vi "Window-Simple Time Series Player.vi"() -> ()   [LabVIEW 2017]
uses:
  User Interface/Visualisation/Timelapse Viewer/Typedefs/Custom slider-vertical.ctl
  User Interface/Visualisation/Timelapse Viewer/Typedefs/Time series viewer refs.ctl
  <vilib>/Utility/miscctls.llb/LVPointTypeDef.ctl
  User Interface/Visualisation/Timelapse Viewer/Typedefs/Speed Viewer States enum.ctl
  Typedefs/Save-Load enum.ctl
  Typedefs/HW config states enum.ctl
  User Interface/Visualisation/Functional Imaging Viewer/Typedefs/Get-Set-Clear Control.ctl
  User Interface/Visualisation/Timelapse Viewer/Typedefs/Select Play-Stop button to show.ctl
  <vilib>/vision/Image Controls.llb/IMAQ Image.ctl
  User Interface/Visualisation/Timelapse Viewer/Globals/gl_Time series viewer globals.vi
  Global Variables/General Globals.vi
panel:
  in  "Intensity":T1={-4095.0, 4095.0} scale=0.0..4095.0
  in  "Back":bool
  in  "Play":bool
  in  "Stop":bool
  in  "Colour":u16(ring)=2 items=["Gray", "Red", "Green"]
  out "Image":T2(plugin-control)
  in  "AVI File Path":path
  out "Speed Graph":dbl[](graph) caption="Speed Chart"
  out "Export data subset":bool
  out "Export vid":bool
  out "Stop (ind)":bool
  in  "Scrollbar":i32(c297)
  out "Speed Profile Graph":dbl[](graph)
  # "<-- Available through the menu"
  # "<-- Available through the menu"
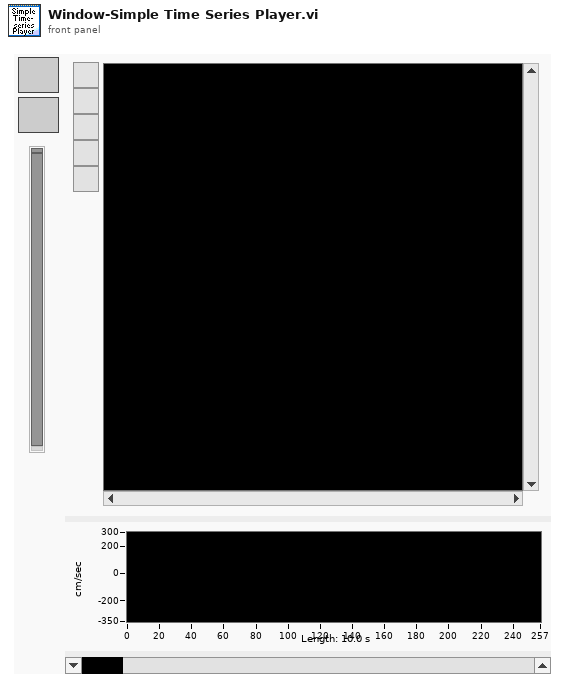
[diagram p1: front panel]
types:
  T1 = typedef "Custom slider-vertical.ctl" = cluster{dbl, dbl}
  T2 = typedef "IMAQ Image.ctl" = refnum<image>
  T3 = typedef "Time series viewer refs.ctl" = cluster{"This VI":refnum<vi>, "Image control":refnum<vi>, "AVI Mode ind":refnum<vi>, "Play":refnum<vi>, "Stop":refnum<vi>, "Back":refnum<vi>, "Scrollbar":refnum<vi>, "Video length info":refnum<vi>, "Expected speed values":refnum<vi>, "Intensity":refnum<vi>, "Path":refnum<vi>, "Selection sliders":refnum<vi>, "Speed Graph ref":refnum<vi>, "Frame rate set (fps)":refnum<vi>, "Channel to load":refnum<vi>, "Number of rows to generate":refnum<vi>, "Colour":refnum<vi>}
  T4 = typedef "LVPointTypeDef.ctl" = cluster{"Horizontal":i16, "Vertical":i16}
  T5 = typedef "HW config states enum.ctl" = enum16{"Load from file", "Save to file", "Write all", "Read all", "Write XY stage settings", "Write DAQ FPGA settings", "Write Control FPGA settings", "Write Phys Channels", "Write System Config", "Write HW Config", "Save System Config", "Save HW Config", "Clear", "Compare from file"}
  T6 = typedef "Save-Load enum.ctl" = enum16{"Save to file", "Load from file", "Compare from file"}
  T7 = typedef "Speed Viewer States enum.ctl" = enum16{"Idle", "Initialise", "Playback", "Scroll bar event", "Speed cursor event", "Back to start", "Exit"}
  T8 = typedef "Image Type" = u32
  T9 = typedef "Custom slider-horisontal.ctl" = cluster{dbl, dbl}
  T10 = typedef "Select Play-Stop button to show.ctl" = enum16{"Show Play button", "Show Stop button"}
  T11 = typedef "AVI modes refs cluster.ctl" = cluster{"AVI1 ref":T12, "AVI2 refs":T13[], "AVI # frames":u32[]}
  T12 = typedef "AviRefnum.ctl" = refnum<k1>
  T13 = typedef "IMAQ AVI2 Refnum.ctl" = refnum<k20>
  T14 = typedef "AVI implementation enum.ctl" = enum16{"AVI1", "AVI2"}
  T15 = cluster{"# of frames to export":i32, "Initial frame's owning file":T13, "8-bit AVI file path":path, "Cursors location":cluster{"Number of first frame":i32, "Number of last frame":i32}}
  T16 = typedef "Get-Set-Clear Control.ctl" = enum16{"Get", "Set", "Clear"}
  T17 = typedef "Speed graph behaviour enum.ctl" = enum16{"Scrolling data", "Scrolling cursor"}
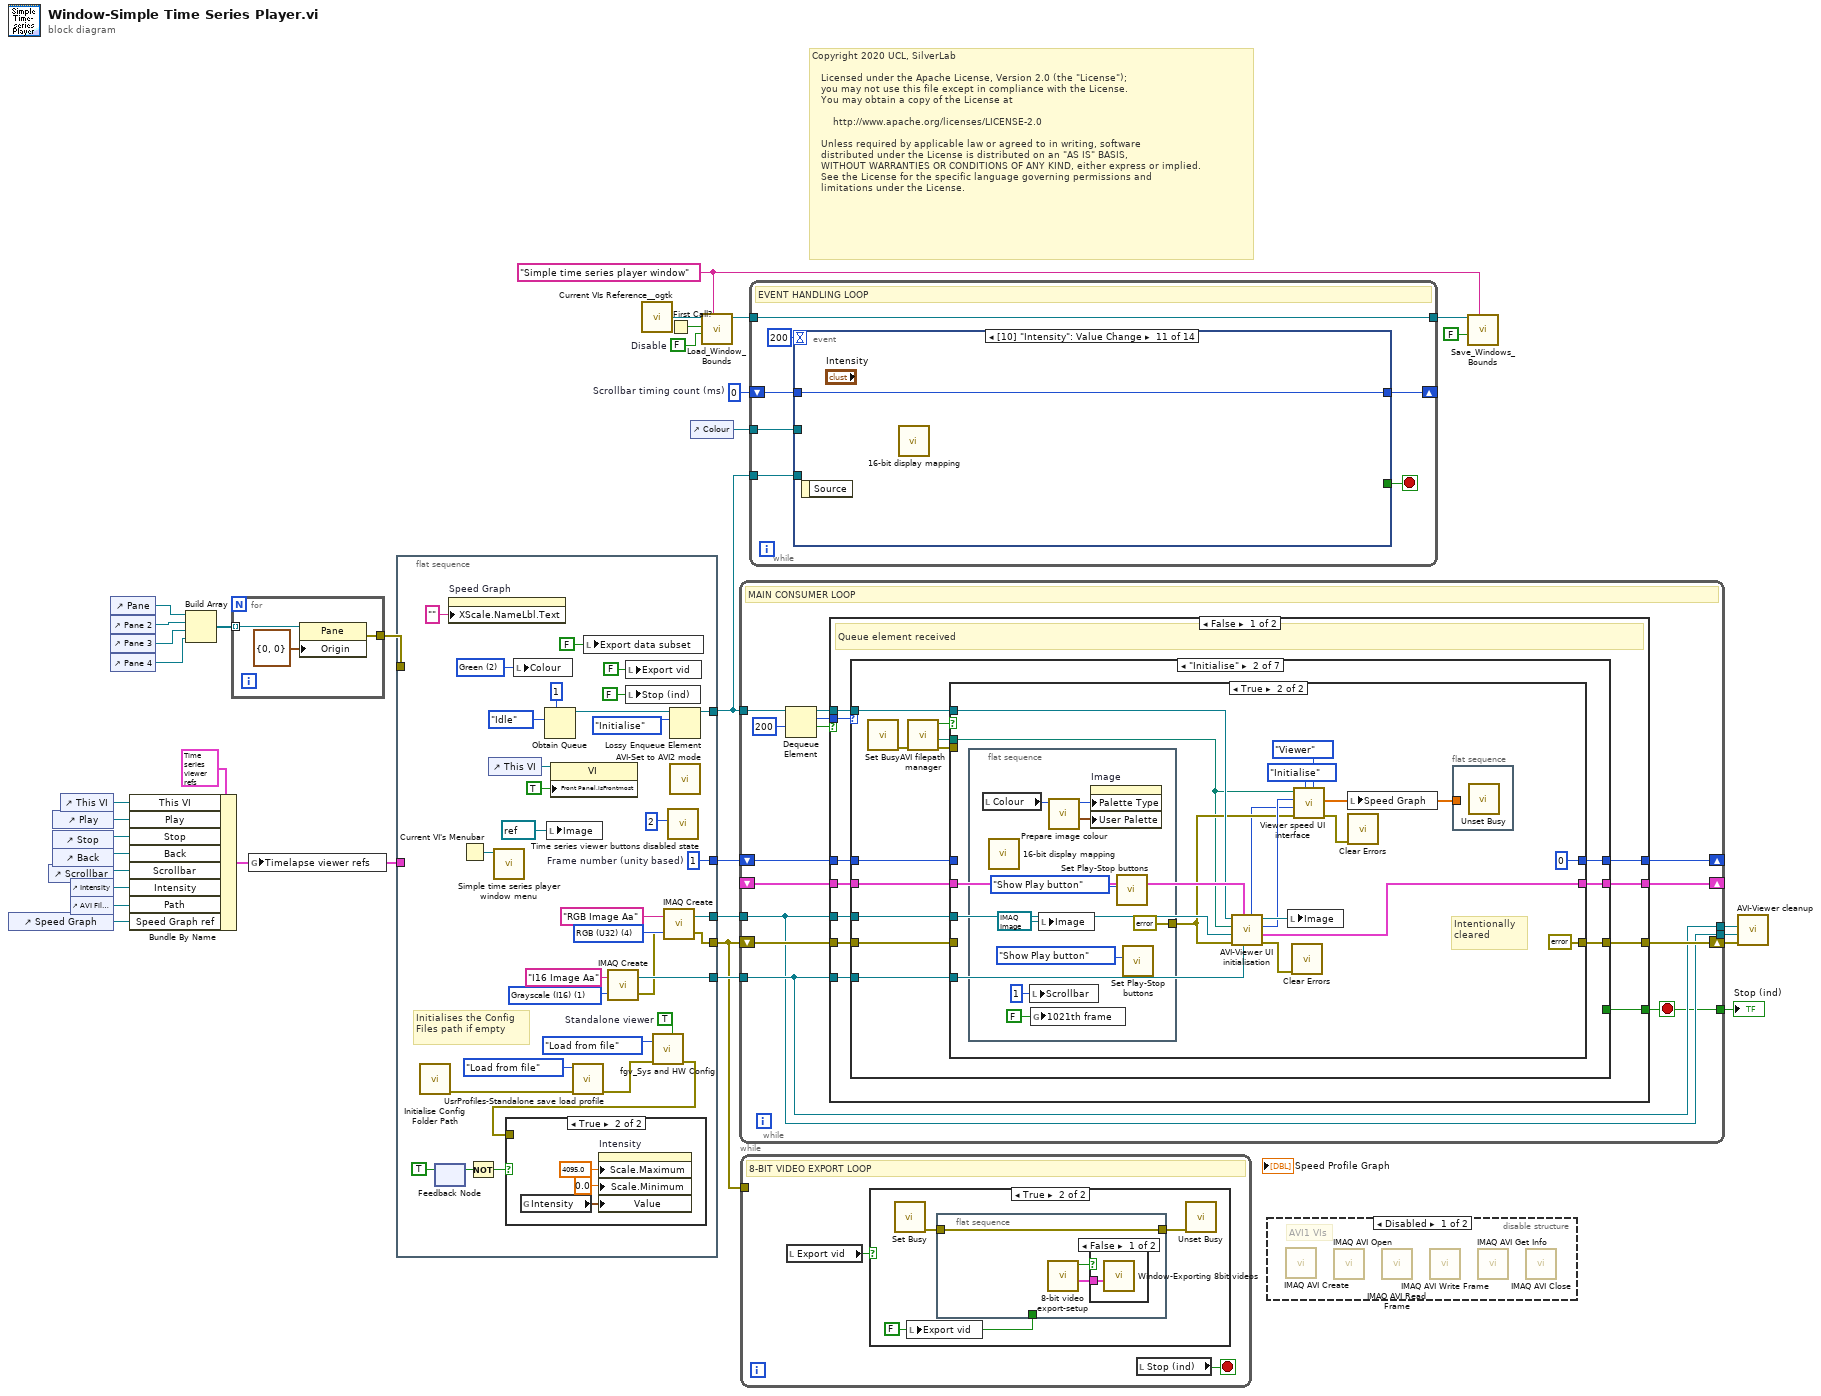
[diagram p0: block diagram]
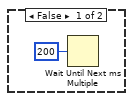
[diagram p3: hidden frame]
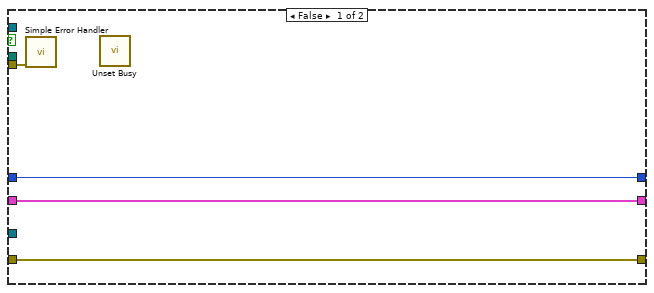
[diagram p7: hidden frame]
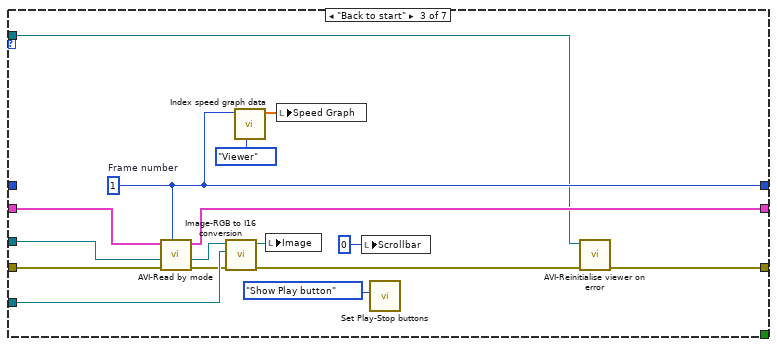
[diagram p8: hidden frame]
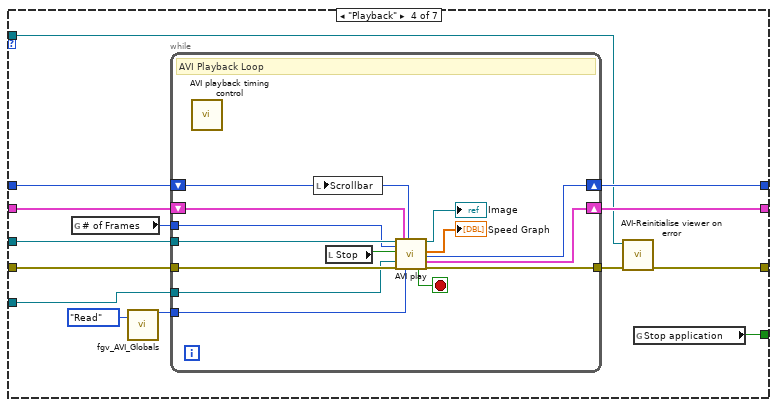
[diagram p9: hidden frame]
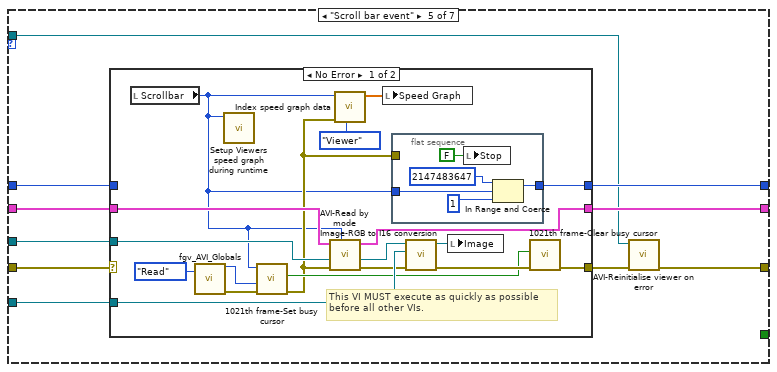
[diagram p10: hidden frame]
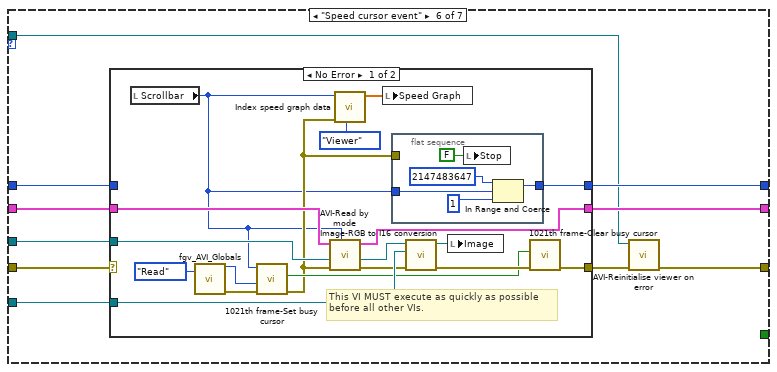
[diagram p12: hidden frame]
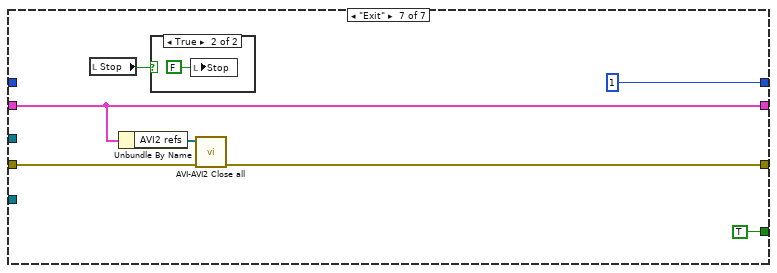
[diagram p14: hidden frame]
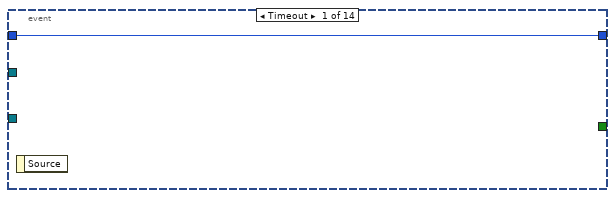
[diagram p17: hidden frame]
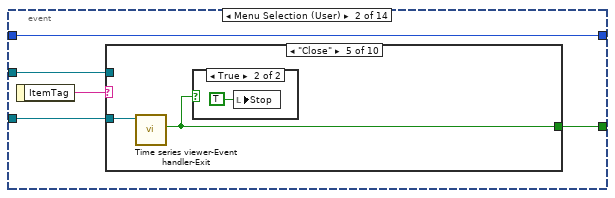
[diagram p18: hidden frame]
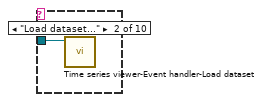
[diagram p20: hidden frame]
diagram:
  w6 = FALSE  # Disable
  w5 = "Simple time series player window" ("Window Name (i.e. Key)")
  w22 = u32 0  # Scrollbar timing count (ms)
  # "Copyright 2020 UCL, SilverLab\n \n   Licensed under the Apache License, Version 2.0 (the \"License\");\n   you may not use this file except in compliance with the License.\n   You may obtain a copy of the License at\n \n       http://www.apache.org/licenses/LICENSE-2.0\n \n   Unless required by applicable law or agreed to in writing, software\n   distributed under the License is distributed on an \"AS IS\" BASIS,\n   WITHOUT WARRANTIES OR CONDITIONS OF ANY KIND, either express or implied.\n   See the License for the specific language governing permissions and\n   limitations under the License."
  n1 = control-ref of="Speed Graph"() -> (w1:refnum<vi>)
  n2 = control-ref of="Scrollbar"() -> (w24:refnum<vi>)
  n3 = control-ref of="Play"() -> (w27:refnum<vi>)
  n4 = control-ref of="Stop"() -> (w26:refnum<vi>)
  n5 = control-ref of="Back"() -> (w25:refnum<vi>)
  n6 = control-ref of="This VI"() -> (w16:refnum<vi>)
  n7 = control-ref of="Intensity"() -> (w23:refnum<vi>)
  n8 = control-ref of="AVI File Path"() -> (w21:refnum<vi>)
  n9 = control-ref of="Pane"() -> (w14:refnum<vi>)
  n10 = control-ref of="Pane 2"() -> (w13:refnum<vi>)
  n11 = control-ref of="Pane 3"() -> (w12:refnum<vi>)
  n12 = control-ref of="Pane 4"() -> (w11:refnum<vi>)
  n13 = Bundle By Name(cluster=T3 {"This VI"=refnum, "Image control"=refnum, "AVI Mode ind"=refnum, "Play"=refnum, "Stop"=refnum, "Back"=refnum, "Scrollbar"=refnum, "Video length info"=refnum, "Expected speed values"=refnum, "Intensity"=refnum, "Path"=refnum, "Selection sliders"=refnum, "Speed Graph ref"=refnum, "Frame rate set (fps)"=refnum, "Channel to load"=refnum, "Number of rows to generate"=refnum, "Colour"=refnum}, "This VI"=w16, "Play"=w27, "Stop"=w26, "Back"=w25, "Scrollbar"=w24, "Intensity"=w23, "Path"=w21, "Speed Graph ref"=w1) -> (w19:T3)
  n14 = Build Array(w14, w13, w12, w11) -> (w10:refnum<vi>[])
  n15 = for {
    tunnel: w10 -> [w36] mode=indexing
    tunnel: [w35] -> w9
    n16 = property class="Pane"(reference=w36, "Origin"=T4 {"Horizontal"=0, "Vertical"=0}) -> (error out=w35:errorcluster)  [unwired: 1 in, 1 out]
  }
  n17 = global write "gl_Time series viewer globals.vi" "Timelapse viewer refs"(w19) -> ()
  n18 = flat-sequence {
    tunnel: [w68] -> w34
    tunnel: [w65] -> w33
    tunnel: [w57] -> w17
    tunnel: [w61] -> w31
    tunnel: [w59] -> w30
    tunnel: w19 -> [_]
    tunnel: w9 -> [_]
    frame #0 {
      w38 = TRUE  # Standalone viewer
      w50 = u16 2 items=["Gray", "Red", "Green"] ("Colour")
      w59 = 1  # Frame number (unity based)
      w67 = T8 1 items=["Grayscale (U8)", "Grayscale (I16)", "Grayscale (SGL)", "Complex (CSG)", "RGB (U32)", "HSL (U32)", "RGB (U64)", "Grayscale (U16)"] ("Image Type")
      w69 = T8 4 items=["Grayscale (U8)", "Grayscale (I16)", "Grayscale (SGL)", "Complex (CSG)", "RGB (U32)", "HSL (U32)", "RGB (U64)", "Grayscale (U16)"] ("Image Type")
      # "Initialises the Config Files path if empty"
      n19 = call "Initialise Config Folder Path.vi"() -> ("error out"=w46:errorcluster)  [unwired: 9 in, 2 out]
      n20 = feedback #1() -> (w43:bool)  [unwired: 1 in]
      n21 = feedback-in #1(TRUE) -> ()
      n22 = property on="Speed Graph" class="WFGraph (strict)"("XScale.NameLbl.Text"="" ("X Scale.Name Label.Text")) -> ()  [unwired: 2 in, 2 out]
      n23 = Current VI's Menubar() -> (w51:refnum<k9>)
      n24 = Not(x=w43) -> (.not. x?=w45:bool)
      n25 = control-ref of="This VI"() -> (w55:refnum<vi>)
      n26 = call "Simple time series player window menu.vi"("menu"=w51) -> ()  [unwired: 9 in, 2 out]
      n27 = local write "Colour"(w50) -> ()
      n28 = Obtain Queue(max queue size (-1, unlimited)=1, element data type=Speed_Viewer_States_enum."Idle" ("States")) -> (queue out=w62:refnum<queue>)  [unwired: 3 in, 2 out]
      n29 = local write "Image"(refnum<image> refnum ("New Image")) -> ()
      n30 = property on="Property Node" class="VI"(reference=w55, "Front Panel.IsFrontmost"=TRUE ("Front Panel Window:Is Frontmost")) -> ()  [unwired: 1 in, 2 out]
      n31 = call "UsrProfiles-Standalone save load profile.vi"("Error in"=w46, "Function"=Save-Load_enum."Load from file") -> ("error out"=w40:errorcluster)  [unwired: 9 in]
      n32 = local write "Export data subset"(FALSE ("Export data subset")) -> ()
      n33 = call "IMAQ Create"("Image Name"="I16 Image Aa", "Image Type"=w67) -> ("New Image"=w65:T2, "error out"=w58:errorcluster)  [unwired: 2 in, 1 out]
      n34 = local write "Export vid"(FALSE ("Export")) -> ()
      n35 = local write "Stop (ind)"(FALSE ("Boolean")) -> ()
      n36 = call "fgv_Sys and HW Config.vi"("Standalone viewer initialisation?"=w38, "Function"=HW_config_states_enum."Load from file", "error in (no error)"=w40) -> ("error out"=w39:errorcluster)  [unwired: 6 in, 2 out]
      n37 = case shown="True" w45 {
        tunnel: w39 -> [_ _]
        frame False {
        }
        frame True {
          n38 = global read "gl_Time series viewer globals.vi" "Intensity"() -> (w71:T9)
          n39 = property on="Intensity" class="Slide (strict)"("Scale.Maximum"=4095.0 ("Scale.Range:Maximum"), "Scale.Minimum"=0.0 ("Scale.Range:Minimum"), "Value"=w71) -> ()  [unwired: 2 in, 2 out]
        }
      }
      n40 = call "IMAQ Create"("Image Name"="RGB Image Aa", "Image Type"=w69, "error in (no error)"=w58) -> ("New Image"=w68:T2, "error out"=w57:errorcluster)  [unwired: 1 in, 1 out]
      n41 = call "Time series viewer buttons disabled state.vi"("Disabled"=2) -> ()  [unwired: 10 in, 1 out]
      n42 = Lossy Enqueue Element(queue=w62, element=Speed_Viewer_States_enum."Initialise" ("States")) -> (queue out=w61:refnum<queue>)  [unwired: 1 in, 3 out]
      n43 = call "AVI-Set to AVI2 mode.vi"() -> ()  [unwired: 11 in, 1 out]
    }
  }
  n44 = call <userlib>:"Current VIs Reference__ogtk.vi"() -> ("Current VI's reference"=w8:refnum<vi>)  [unwired: 5 in]
  n45 = First Call?() -> (First Call?: T/F=w7:bool)
  n46 = control-ref of="Colour"() -> (w15:refnum<vi>)
  n47 = call "Load_Window_Bounds.vi"("Window Name (i.e. Key)"=w5, "Disable"=w6, "First Call"=w7, "Window VI's Ref"=w8) -> ("reference out"=w3:refnum<vi>)  [unwired: 4 in, 3 out]
  n48 = while {
    tunnel: w34 -> [w76]
    tunnel: w33 -> [w77]
    tunnel: [w77] -> w32
    shift-right: [w84] -> _
    shift-left: w30 -> [w83]
    tunnel: w31 -> [w82]
    shift-right: [w78] -> _
    shift-left: _ -> [w87]
    tunnel: [w76] -> w20
    shift-right: [w85] -> w28
    shift-left: w17 -> [w86]
    tunnel: [w74] -> w18
    stop <- w74 stop-if-true
    # "MAIN CONSUMER LOOP"
    n49 = Dequeue Element(queue=w82, timeout in ms (-1)=200) -> (queue out=w75:refnum<queue>, element=w79:T7, timed out?=w80:bool)  [unwired: 1 in, 1 out]
    n50 = case shown="False" w80 {
      tunnel: w87 -> [w98 w270]
      tunnel: [w97 w270] -> w78
      tunnel: w76 -> [w96 _]
      tunnel: w77 -> [w95 _]
      tunnel: w86 -> [w94 w269]
      tunnel: [w93 w269] -> w85
      tunnel: [w92 w271] -> w84
      tunnel: w83 -> [w91 w271]
      tunnel: w79 -> [w90 _]
      tunnel: [w89 _] -> w74
      tunnel: w75 -> [w88 _]
      frame False {
        # "Queue element received"
        n51 = case shown="\"Initialise\"" w90 {
          tunnel: w98 -> [w100 w114 w158 w174 w194 w230 w263]
          tunnel: [w100 w110 w157 w168 w196 w232 w263] -> w97
          tunnel: w96 -> [_ w109 w155 w173 w195 w231 _]
          tunnel: w95 -> [_ w108 w156 w172 w198 w234 _]
          tunnel: w94 -> [w99 w112 w153 w171 w193 w229 w262]
          tunnel: [w99 w111 w148 w167 w191 w227 w261] -> w93
          tunnel: [w101 w113 w150 w170 w197 w233 1 ("Slide")] -> w92
          tunnel: w91 -> [w101 w107 _ w169 w192 w228 _]
          tunnel: [_ _ _ w161 _ _ TRUE] -> w89
          tunnel: w88 -> [_ w103 w147 w165 w189 w225 _]
          frame Default {
          }
          frame "Initialise" {
            n52 = call <vilib>:"Set Busy.vi"() -> ("error out"=w102:errorcluster)  [unwired: 10 in, 1 out]
            n53 = call "AVI filepath manager.vi"("error in (no error)"=w102) -> ("error"=w104:errorcluster, "AVI File Path"=w105:path, "File path OK"=w106:bool)  [unwired: 8 in]
            n54 = case shown="True" w106 {
              tunnel: w114 -> [w117 w135]
              tunnel: [w118 0] -> w113
              tunnel: w105 -> [_ w125]
              tunnel: w112 -> [w116 _]
              tunnel: [w116 errorcluster {"status"=FALSE, "code"=0, "source"=""} ("error out")] -> w111
              tunnel: [w117 w128] -> w110
              tunnel: w109 -> [_ w127]
              tunnel: w108 -> [_ w133]
              tunnel: w107 -> [w118 _]
              tunnel: w104 -> [w115 _]
              tunnel: w103 -> [_ w131]
              frame False {
                n55 = call <vilib>:"Simple Error Handler.vi"("error in (no error)"=w115) -> ()  [unwired: 4 in, 5 out]
                n56 = call <vilib>:"Unset Busy.vi"() -> ()  [unwired: 11 in, 1 out]
              }
              frame True {
                # "Intentionally cleared"
                n57 = flat-sequence {
                  tunnel: [errorcluster {"status"=FALSE, "code"=0, "source"=""} ("error out")] -> w126
                  frame #0 {
                    n58 = local read "Colour"() -> (w139:u16)
                    n59 = call "16-bit display mapping.vi"() -> ()  [unwired: 11 in, 1 out]
                    n60 = local write "Scrollbar"(1 ("Scrollbar")) -> ()
                    n61 = global write "gl_Time series viewer globals.vi" "1021th frame"(FALSE ("1021th frame")) -> ()
                    n62 = local write "Image"(T2 refnum ("New Image")) -> ()
                    n63 = call "Prepare image colour.vi"("Left Image Palette"=w139) -> ("Color Palette"=w141:cluster{"Red":u8, "Green":u8, "Blue":u8}[], "Palette Type"=w140:u32)  [unwired: 8 in, 1 out]
                    n64 = property on="Image" class="ImageControl"("Palette Type"=w140, "User Palette"=w141) -> ()  [unwired: 2 in, 2 out]
                    n65 = call "Set Play-Stop buttons.vi"("Function"=Select_Play-Stop_button_to_show."Show Play button") -> ()  [unwired: 10 in, 1 out]
                    n66 = call "Set Play-Stop buttons.vi"("Function"=Select_Play-Stop_button_to_show."Show Play button") -> ()  [unwired: 10 in, 1 out]
                  }
                }
                n67 = call "AVI-Viewer UI initialisation.vi"("I16 image ref in"=w133, "AVI modes refs in"=w135, "error in (no error)"=w126, "RGB image ref in"=w127, "AVI File Path"=w125, "Queue in"=w131) -> ("error out"=w120:errorcluster, "AVI modes refs out"=w128:T11, "Number of Frames"=w129:u32, "Refnum out"=w130:T2, "Scrollbar position"=w122:i32)  [unwired: 1 in]
                n68 = local write "Image"(w130) -> ()
                n69 = call <vilib>:"Clear Errors.vi"("error in (no error)"=w120) -> ()  [unwired: 5 in, 2 out]
                n70 = call "Viewer speed UI interface.vi"("Caller"=enum16{"Viewer", "Exporter"}."Viewer", "Function"=enum16{"Initialise", "Update"}."Initialise", "error in (no error)"=w126, "Gobal frame number in Timelapse data/master video (1 based)"=w122, "Number of Frames"=w129, "Speed Data folder path+dummy filename"=w125) -> ("error out"=w124:errorcluster, "Speed waveform graph data"=w119:dbl[])  [unwired: 2 in, 2 out]
                n71 = local write "Speed Graph"(w119) -> ()
                n72 = call <vilib>:"Clear Errors.vi"("error in (no error)"=w124) -> ()  [unwired: 5 in, 2 out]
                n73 = flat-sequence {
                  tunnel: w119 -> [_]
                  frame #0 {
                    n74 = call <vilib>:"Unset Busy.vi"() -> ()  [unwired: 11 in, 1 out]
                  }
                }
              }
            }
          }
          frame "Back to start" {
            w150 = 1  # Frame number
            n75 = call "AVI-Read by mode.vi"("Frame number (unity-based)"=w150, "error in (no error)"=w153, "RGB image ref in"=w155, "AVI modes refs"=w158) -> ("error out"=w152:errorcluster, "RGB image ref out"=w159:T2, "AVI modes refs"=w157:T11)  [unwired: 5 in]
            n76 = call "Image-RGB to I16 conversion.vi"("error in (no error)"=w152, "I16 image ref in"=w156, "RGB image ref in"=w159) -> ("error out"=w149:errorcluster, "I16 image ref out"=w154:T2)  [unwired: 7 in]
            n77 = call "Index speed graph data.vi"("Caller"=enum16{"Viewer", "Exporter"}."Viewer", "Gobal frame number in Timelapse data/master video (1 based)"=w150) -> ("Speed data waveform graph"=w145:dbl[])  [unwired: 7 in, 2 out]
            n78 = local write "Image"(w154) -> ()
            n79 = local write "Speed Graph"(w145) -> ()
            n80 = local write "Scrollbar"(0 ("Scrollbar")) -> ()
            n81 = call "Set Play-Stop buttons.vi"("Function"=Select_Play-Stop_button_to_show."Show Play button") -> ()  [unwired: 10 in, 1 out]
            n82 = call "AVI-Reinitialise viewer on error.vi"("error in (no error)"=w149, "Queue in"=w147) -> ("error out"=w148:errorcluster)  [unwired: 9 in]
          }
          frame "Playback" {
            n83 = global read "gl_Time series viewer globals.vi" "# of Frames"() -> (w162:u32)
            n84 = call "fgv_AVI_Globals.vi"("Function"=enum16{"Intialize", "Write", "Read", "Clear"}."Read") -> ("AVI mode"=w163:T14)  [unwired: 11 in, 3 out]
            n85 = while {
              tunnel: w173 -> [w186]
              tunnel: w172 -> [w178]
              tunnel: w171 -> [w184]
              tunnel: [w185] -> w166
              shift-right: [w182] -> w170
              shift-left: w169 -> [w183]
              shift-right: [w187] -> w168
              shift-left: w174 -> [w188]
              tunnel: w163 -> [w180]
              tunnel: w162 -> [w177]
              stop <- w181 stop-if-true
              # "AVI Playback Loop"
              n86 = call "AVI playback timing control.vi"() -> ()  [unwired: 8 in, 4 out]
              n87 = local write "Scrollbar"(w183) -> ()
              n88 = local read "Stop"() -> (w179:bool)
              n89 = call "AVI play.vi"("RGB Image ref"=w186, "Number of Frames"=w177, "Stop button pressed"=w179, "I16 Image ref"=w178, "error in (no error)"=w184, "AVI modes refs in"=w188, "AVI mode"=w180, "Frame number (in)"=w183) -> ("Playback stopped"=w181:bool, "I16 image ref out"=→"Image":T2, "Speed data waveform graph"=→"Speed Graph":dbl[], "Frame number (out)"=w182:i32, "AVI modes refs out"=w187:T11, "error out"=w185:errorcluster)  [unwired: 6 in]
            }
            n90 = call "AVI-Reinitialise viewer on error.vi"("error in (no error)"=w166, "Queue in"=w165) -> ("error out"=w167:errorcluster)  [unwired: 9 in]
            n91 = global read "General Globals.vi" "Stop application"() -> (w161:bool)
          }
          frame "Scroll bar event" {
            n92 = case shown="No Error" w193 {
              selector: w193 -> [_ w224]
              tunnel: w198 -> [w216 _]
              tunnel: [w214 w223] -> w197
              tunnel: [w203 w222] -> w196
              tunnel: w195 -> [w212 _]
              tunnel: w194 -> [w210 w222]
              tunnel: [w205 w224] -> w190
              tunnel: w192 -> [_ w223]
              frame No Error {
                # "This VI MUST execute as quickly as possible\nbefore all other VIs."
                n93 = local read "Scrollbar"() -> (w199:i32)
                n94 = call "fgv_AVI_Globals.vi"("Function"=enum16{"Intialize", "Write", "Read", "Clear"}."Read") -> ("AVI mode"=w208:T14, "error out"=w207:errorcluster)  [unwired: 11 in, 2 out]
                n95 = call "Setup Viewers speed graph during runtime.vi"("Frame number or cycle number"=w199) -> ()  [unwired: 10 in, 1 out]
                n96 = call "1021th frame-Set busy cursor.vi"("error in (no error)"=w207, "AVI mode"=w208, "Frame number"=w199) -> ("error out"=w202:errorcluster, "Busy cursor was set"=w204:bool)  [unwired: 7 in]
                n97 = call "AVI-Read by mode.vi"("Frame number (unity-based)"=w199, "error in (no error)"=w202, "RGB image ref in"=w212, "AVI modes refs"=w210) -> ("error out"=w213:errorcluster, "RGB image ref out"=w211:T2, "AVI modes refs"=w203:T11)  [unwired: 5 in]
                n98 = call "Index speed graph data.vi"("Caller"=enum16{"Viewer", "Exporter"}."Viewer", "error in (no error)"=w202, "Gobal frame number in Timelapse data/master video (1 based)"=w199) -> ("Speed data waveform graph"=w200:dbl[])  [unwired: 6 in, 2 out]
                n99 = local write "Speed Graph"(w200) -> ()
                n100 = flat-sequence {
                  tunnel: [w219] -> w214
                  tunnel: w199 -> [w217]
                  tunnel: w202 -> [_]
                  frame #0 {
                    n101 = local write "Stop"(FALSE ("Stop")) -> ()
                    n102 = In Range and Coerce(upper limit=2147483647, x=w217, lower limit=1) -> (coerced(x)=w219:i32)  [unwired: 1 out]
                  }
                }
                n103 = call "Image-RGB to I16 conversion.vi"("error in (no error)"=w213, "I16 image ref in"=w216, "RGB image ref in"=w211) -> ("error out"=w206:errorcluster, "I16 image ref out"=w215:T2)  [unwired: 7 in]
                n104 = local write "Image"(w215) -> ()
                n105 = call "1021th frame-Clear busy cursor.vi"("error in (no error)"=w206, "Busy cursor was set"=w204) -> ("error out"=w205:errorcluster)  [unwired: 9 in]
              }
              frame Error {
              }
            }
            n106 = call "AVI-Reinitialise viewer on error.vi"("error in (no error)"=w190, "Queue in"=w189) -> ("error out"=w191:errorcluster)  [unwired: 9 in]
          }
          frame "Speed cursor event" {
            n107 = case shown="No Error" w229 {
              selector: w229 -> [_ w260]
              tunnel: w234 -> [w252 _]
              tunnel: [w250 w259] -> w233
              tunnel: [w239 w258] -> w232
              tunnel: w231 -> [w248 _]
              tunnel: w230 -> [w246 w258]
              tunnel: [w241 w260] -> w226
              tunnel: w228 -> [_ w259]
              frame No Error {
                # "This VI MUST execute as quickly as possible\nbefore all other VIs."
                n108 = local read "Scrollbar"() -> (w235:i32)
                n109 = call "fgv_AVI_Globals.vi"("Function"=enum16{"Intialize", "Write", "Read", "Clear"}."Read") -> ("AVI mode"=w244:T14, "error out"=w243:errorcluster)  [unwired: 11 in, 2 out]
                n110 = call "1021th frame-Set busy cursor.vi"("error in (no error)"=w243, "AVI mode"=w244, "Frame number"=w235) -> ("error out"=w238:errorcluster, "Busy cursor was set"=w240:bool)  [unwired: 7 in]
                n111 = call "AVI-Read by mode.vi"("Frame number (unity-based)"=w235, "error in (no error)"=w238, "RGB image ref in"=w248, "AVI modes refs"=w246) -> ("error out"=w249:errorcluster, "RGB image ref out"=w247:T2, "AVI modes refs"=w239:T11)  [unwired: 5 in]
                n112 = call "Index speed graph data.vi"("Caller"=enum16{"Viewer", "Exporter"}."Viewer", "error in (no error)"=w238, "Gobal frame number in Timelapse data/master video (1 based)"=w235) -> ("Speed data waveform graph"=w236:dbl[])  [unwired: 6 in, 2 out]
                n113 = local write "Speed Graph"(w236) -> ()
                n114 = flat-sequence {
                  tunnel: [w255] -> w250
                  tunnel: w235 -> [w253]
                  tunnel: w238 -> [_]
                  frame #0 {
                    n115 = local write "Stop"(FALSE ("Stop")) -> ()
                    n116 = In Range and Coerce(upper limit=2147483647, x=w253, lower limit=1) -> (coerced(x)=w255:i32)  [unwired: 1 out]
                  }
                }
                n117 = call "Image-RGB to I16 conversion.vi"("error in (no error)"=w249, "I16 image ref in"=w252, "RGB image ref in"=w247) -> ("error out"=w242:errorcluster, "I16 image ref out"=w251:T2)  [unwired: 7 in]
                n118 = local write "Image"(w251) -> ()
                n119 = call "1021th frame-Clear busy cursor.vi"("error in (no error)"=w242, "Busy cursor was set"=w240) -> ("error out"=w241:errorcluster)  [unwired: 9 in]
              }
              frame Error {
              }
            }
            n120 = call "AVI-Reinitialise viewer on error.vi"("error in (no error)"=w226, "Queue in"=w225) -> ("error out"=w227:errorcluster)  [unwired: 9 in]
          }
          frame "Exit" {
            n121 = local read "Stop"() -> (w267:bool)
            n122 = Unbundle By Name(w263) -> ("AVI2 refs"=w264:T13[])
            n123 = case shown="True" w267 {
              frame False {
              }
              frame True {
                n124 = local write "Stop"(FALSE ("Stop")) -> ()
              }
            }
            n125 = call "AVI-AVI2 Close all.vi"("error in (no error)"=w262, "AVI2 ref"=w264) -> ("error out"=w261:errorcluster)  [unwired: 9 in]
          }
        }
      }
      frame True {
        # "Timeout"
      }
    }
  }
  "Stop (ind)" <- w18
  n126 = while {
    tunnel: w17 -> [_]
    stop <- w273 stop-if-true
    # "8-BIT VIDEO EXPORT LOOP"
    n127 = local read "Export vid"() -> (w272:bool)
    n128 = case shown="True" w272 {
      frame False {
        n129 = Wait Until Next ms Multiple(millisecond multiple=u32 200) -> ()  [unwired: 1 out]
      }
      frame True {
        w277 = FALSE ("Export")
        n130 = call <vilib>:"Set Busy.vi"() -> ("error out"=w276:errorcluster)  [unwired: 10 in, 1 out]
        n131 = local write "Export vid"(w277) -> ()
        n132 = flat-sequence {
          tunnel: w277 -> [_]
          tunnel: w276 -> [w280]
          tunnel: [w280] -> w275
          frame #0 {
            n133 = call "8-bit video export-setup.vi"() -> ("output cluster"=w278:T15, "cancelled"=w279:bool)  [unwired: 9 in, 1 out]
            n134 = case shown="False" w279 {
              tunnel: w278 -> [w281 _]
              frame False {
                n135 = call "Window-Exporting 8bit videos.vi"("Input cluster"=w281) -> ()  [unwired: 11 in]
              }
              frame True {
              }
            }
          }
        }
        n136 = call <vilib>:"Unset Busy.vi"("error in (no error)"=w275) -> ()  [unwired: 10 in, 1 out]
      }
    }
    n137 = local read "Stop (ind)"() -> (w273:bool)
  }
  n138 = while {
    shift-right: [w286] -> _
    shift-left: w22 -> [w285]
    tunnel: w31 -> [w284]
    tunnel: w15 -> [w283]
    tunnel: [w282] -> w2
    tunnel: w3 -> [w282]
    stop <- w287 stop-if-true
    # "EVENT HANDLING LOOP"
    n139 = event shown="[10] \"Intensity\": Value Change" {
      selector: _ -> [_ _ _ _ _ _ _ _ _ _ _ _ _ _]
      dyn-events: _ -> [_ _ _ _ _ _ _ _ _ _ _ _ _ _]
      timeout: 200 -> [_ _ _ _ _ _ _ _ _ _ _ _ _ _]
      tunnel: [_ w291 _ _ _ _ _ _ _ _ _ _ _ w360] -> w287
      tunnel: [w289 w294 w309 w310 w318 w326 w330 w336 w339 w345 w346 w350 w358 w362] -> w286
      tunnel: w285 -> [w289 w294 w309 w312 w318 w326 w330 w336 w339 w345 w346 w350 w358 w362]
      tunnel: w284 -> [_ w292 _ w311 _ w324 _ _ w338 w342 _ w349 _ w361]
      tunnel: w283 -> [_ w290 _ _ _ _ _ _ _ _ _ _ _ _]
      event Timeout {
        n140 = event-data() -> ()  [unwired: 1 in, 1 out]
      }
      event Menu Selection (User) {
        n141 = event-data() -> ("ItemTag"=w293:string)  [unwired: 1 in]
        n142 = case shown="\"Close\"" w293 {
          tunnel: w292 -> [_ w295 _ _ w298 _ _ _ _ _]
          tunnel: [_ _ _ _ w297 _ _ _ _ _] -> w291
          tunnel: w290 -> [_ _ _ _ _ _ _ w303 w305 w307]
          frame Default {
          }
          frame "Load dataset..." {
            n143 = call "Time series viewer-Event handler-Load dataset.vi"("queue"=w295) -> ()  [unwired: 11 in]
          }
          frame "Playback speed..." {
            n144 = call "Window-Playback speed entry.vi"() -> ()  [unwired: 10 in, 2 out]
          }
          frame "Original speed (x1)" {
            n145 = flat-sequence {
              frame #0 {
                n146 = global write "gl_Time series viewer globals.vi" "Use manual FPS?"(FALSE ("Use manual FPS?")) -> ()
              }
              frame #1 {
                n147 = call "AVI playback timing control.vi"() -> ()  [unwired: 8 in, 4 out]
              }
            }
          }
          frame "Close" {
            n148 = call "Time series viewer-Event handler-Exit.vi"("Queue in"=w298) -> ("Exit"=w297:bool)  [unwired: 10 in]
            n149 = case shown="True" w297 {
              frame False {
              }
              frame True {
                n150 = local write "Stop"(TRUE ("Stop")) -> ()
              }
            }
          }
          frame "Export 8-bit video file..." {
            "Export vid" <- TRUE
          }
          frame "Export time-lapse subset..." {
            "Export data subset" <- TRUE
          }
          frame "Red" {
            w302 = u16 1 items=["Gray", "Red", "Green"] ("Colour")
            n151 = property class="Ring (strict)"(reference=w303, "Val(Sgnl)"=w302) -> ()  [unwired: 1 in, 2 out]
          }
          frame "Green" {
            w304 = u16 2 items=["Gray", "Red", "Green"] ("Colour")
            n152 = property class="Ring (strict)"(reference=w305, "Val(Sgnl)"=w304) -> ()  [unwired: 1 in, 2 out]
          }
          frame "Gray" {
            w306 = u16 0 items=["Gray", "Red", "Green"] ("Colour")
            n153 = property class="Ring (strict)"(reference=w307, "Val(Sgnl)"=w306) -> ()  [unwired: 1 in, 2 out]
          }
        }
      }
      event "Scrollbar", "Speed Graph": Shortcut Menu Selection (User) {
        n154 = event-data() -> ("ItemTag"=w308:string)  [unwired: 1 in]
        n155 = call "Time series viewer-Shortcut menu handler.vi"("ItemTag"=w308) -> ()  [unwired: 11 in]
      }
      event "Scrollbar": Value Change {
        n156 = event-data() -> ()  [unwired: 1 in, 1 out]
        n157 = call "Event case-Scrollbar value change.vi"("Tick count in"=w312, "Queue in"=w311) -> ("Tick count"=w310:u32)  [unwired: 8 in, 1 out]
      }
      event "Speed Graph": Shortcut Menu Activation? {
        n158 = event-data() -> ("MenuRef"=w313:refnum<k9>)  [unwired: 1 in]
        n159 = call "FGV_Speed graph behaviour-Main viewer.vi"("Function"=Get-Set-Clear_Control."Get") -> ("Speed graph behaviour"=w315:T17)  [unwired: 9 in, 1 out]
        n160 = case shown="\"Scrolling data\", Default" w315 {
          tunnel: [bool[] [FALSE, TRUE] bool[] [TRUE, FALSE]] -> w314
          frame "Scrolling data", Default {
          }
          frame "Scrolling cursor" {
          }
        }
        n161 = for {
          tunnel: string[] ["scrolling cursor", "scrolling data"] -> [w323] mode=indexing
          tunnel: w313 -> [w322]
          tunnel: w314 -> [w321] mode=indexing
          n162 = Set Menu Item Info(6:w321, 7:w323, 11:w322) -> ()  [unwired: 4 in, 2 out]
        }
        n163 = event-data() -> ()  [unwired: 2 in, 1 out]
      }
      event "Speed Graph": Cursor Move; "Speed Graph": Cursor Release {
        n164 = event-data() -> ("CursRef"=w325:refnum<vi>)  [unwired: 1 in]
        n165 = call "Event case-Speed graph cursor moved.vi"("queue in"=w324, "Cursor in"=w325) -> ()  [unwired: 9 in, 1 out]
      }
      event "Speed Graph": event type 3.0.x80000027 {
        n166 = event-data() -> ()  [unwired: 1 in, 1 out]
        n167 = call "FGV_Speed graph behaviour-Main viewer.vi"("Function"=Get-Set-Clear_Control."Get") -> ("Speed graph behaviour"=w329:T17)  [unwired: 9 in, 1 out]
        n168 = case shown="\"Scrolling data\", Default" w329 {
          tunnel: [TRUE FALSE] -> w327
          frame "Scrolling data", Default {
            # "Moving the speed data graph's cursor manually is \nprevented when the mode is \"Scrolling data\"."
          }
          frame "Scrolling cursor" {
            # "Moving the speed data graph's cursor manually is \nallowed when the mode is \"Scrolling cursor\"."
          }
        }
        n169 = event-data("Discard?"=w327) -> ()  [unwired: 1 in, 1 out]
      }
      event "Colour": Value Change {
        n170 = event-data() -> ()  [unwired: 1 in, 1 out]
        n171 = call "Prepare image colour.vi"("Left Image Palette"="Colour") -> ("Color Palette"=w333:cluster{"Red":u8, "Green":u8, "Blue":u8}[], "Palette Type"=w334:u32)  [unwired: 8 in, 1 out]
        n172 = property on="Image" class="ImageControl"("Palette Type"=w334, "User Palette"=w333) -> ()  [unwired: 2 in, 2 out]
      }
      event "AVI File Path": Value Change {
        w337 = TRUE ("Stop")
        n173 = event-data() -> ()  [unwired: 1 in, 1 out]
        n174 = local write "Stop"(w337) -> ()
        n175 = flat-sequence {
          tunnel: w338 -> [w341]
          tunnel: w337 -> [_]
          frame #0 {
            n176 = Enqueue Element At Opposite End(queue=w341, element=Speed_Viewer_States_enum."Initialise") -> ()  [unwired: 2 in, 3 out]
          }
        }
      }
      event "Back": Value Change {
        n177 = event-data() -> ()  [unwired: 1 in, 1 out]
        n178 = Enqueue Element At Opposite End(queue=w342, element=Speed_Viewer_States_enum."Back to start") -> ()  [unwired: 2 in, 3 out]
        n179 = local write "Stop"(TRUE ("Stop")) -> ()
      }
      event Value Change {
        n180 = event-data() -> ()  [unwired: 1 in, 1 out]
        n181 = call "16-bit display mapping.vi"() -> ()  [unwired: 11 in, 1 out]
      }
      event "Play": Value Change {
        n182 = event-data() -> ()  [unwired: 1 in, 1 out]
        n183 = flat-sequence {
          tunnel: w349 -> [w354]
          tunnel: [w354] -> w348
          tunnel: w348 -> [w355]
          tunnel: [w355] -> w347
          tunnel: w347 -> [w356]
          frame #0 {
            n184 = property on="Speed Graph" class="WFGraph (strict)"("Value"=dbl[] [] ("History Data")) -> ()  [unwired: 2 in, 2 out]
            n185 = local write "Stop"(FALSE ("Stop")) -> ()
            n186 = call "Set Play-Stop buttons.vi"("Function"=Select_Play-Stop_button_to_show."Show Stop button") -> ()  [unwired: 10 in, 1 out]
          }
          frame #1 {
            n187 = call "Set scrollbar at start.vi"("Queue in"=w355) -> ()  [unwired: 10 in, 1 out]
          }
          frame #2 {
            n188 = Enqueue Element(queue=w356, element=Speed_Viewer_States_enum."Playback" ("States")) -> ()  [unwired: 2 in, 3 out]
          }
        }
      }
      event "Stop": Value Change {
        n189 = event-data() -> ()  [unwired: 1 in, 1 out]
      }
      event Panel Close? {
        n190 = event-data() -> ()  [unwired: 1 in, 1 out]
        n191 = call "Time series viewer-Event handler-Exit.vi"("Queue in"=w361) -> ("Exit"=w360:bool)  [unwired: 10 in]
        n192 = case shown="True" w360 {
          frame False {
          }
          frame True {
            n193 = local write "Stop"(TRUE ("Stop")) -> ()
          }
        }
        n194 = event-data("Discard?"=TRUE) -> ()  [unwired: 1 in, 1 out]
      }
    }
  }
  n195 = disable-structure shown="Disabled" {
    frame Disabled {
      # "AVI1 VIs"
      n196 = call "IMAQ AVI Create"() -> ()  [unwired: 10 in, 2 out]
      n197 = call "IMAQ AVI Open"() -> ()  [unwired: 10 in, 2 out]
      n198 = call "IMAQ AVI Read Frame"() -> ()  [unwired: 8 in, 4 out]
      n199 = call "IMAQ AVI Write Frame"() -> ()  [unwired: 10 in, 2 out]
      n200 = call "IMAQ AVI Get Info"() -> ()  [unwired: 7 in, 5 out]
      n201 = call "IMAQ AVI Close"() -> ()  [unwired: 11 in, 1 out]
    }
    frame Enabled {
    }
  }
  n202 = call "Save_Windows_Bounds.vi"("Window Name (i.e. Key)"=w5, "Front Panel Window:Open"=FALSE, "Window VI's Ref"=w2) -> ()  [unwired: 8 in, 1 out]
  n203 = call "AVI-Viewer cleanup.vi"("error in (no error)"=w28, "RGB image ref"=w20, "I16 image ref"=w32) -> ()  [unwired: 8 in, 1 out]
